vi "all filters coeffs.vi"(9 "taps diff":i32=17, 10 "sampling freq: fs":dbl=110250.0 min=-1e-308 max=1e+308 format="%0.2f", 11 "?":T2={"Amplitude"=1.0, "Lower Freq"=0.0, "Higher Freq"=25000.0, "Weighted\nRipple"=1e-06} {"Weighted\nRipple" min=-1e-308 max=1e+308 format="%0.2e"; "Higher Freq" min=-1e-308 max=1e+308 format="%0.2f"; "Lower Freq" min=-1e-308 max=1e+308 format="%0.2f"; "Amplitude" min=-1e-308 max=1e+308 format="%0.2f"}) -> (1 "ripple diff":dbl format="%0.2f", 2 "diff":dbl[](array[numeric])=[-1.090529051367417e-05, 0.00012379655057511986, -0.0007235759415153059, 0.0028997025258309344, -0.00899855784923205, 0.023414742171632856, -0.055622216670635403, 0.14563551285330884, 0.0, -0.14563551285330884, 0.055622216670635403, -0.023414742171632856, 0.00899855784923205, -0.0028997025258309344, 0.0007235759415153059, -0.00012379655057511986, 1.090529051367417e-05])   [LabVIEW 2017]
uses:
  <vilib>/Analysis/2dsp.llb/Real FFT.vi
  <vilib>/Analysis/3filter.llb/FIR Filter (DBL).vi
  <vilib>/Analysis/NI_AALBase.lvlib
  <vilib>/Analysis/NI_AALPro.lvlib
panel:
  in  "Tab Control":T1(tab)
  in  "?":T2={"Amplitude"=1.0, "Lower Freq"=1000.0, "Higher Freq"=49000.0, "Weighted\nRipple"=0.001} {"Weighted\nRipple" min=-1e-308 max=1e+308 format="%0.2e"; "Higher Freq" min=-1e-308 max=1e+308 format="%0.2f"; "Lower Freq" min=-1e-308 max=1e+308 format="%0.2f"; "Amplitude" min=-1e-308 max=1e+308 format="%0.2f"}
  in  "taps hilbert":i32=33
  in  "sampling freq: fs 2":dbl=110250.0 min=-1e-308 max=1e+308 format="%0.2f"
  out "hilbert":dbl[](graph)
  out "ripple hilbert":dbl format="%0.2f"
  out "hilbert":dbl[](array[numeric])
  out "K(omega) 2":dbl[](graph)
  out "diff":dbl[](graph)
  out "K(omega)":dbl[](graph)
  in  "demp":dbl=0.7
  in  "Fr":dbl=12000.0
  out "g1":dbl
  out "g2":dbl
  in  "discr freq":dbl=110250.0
  out "error":i32
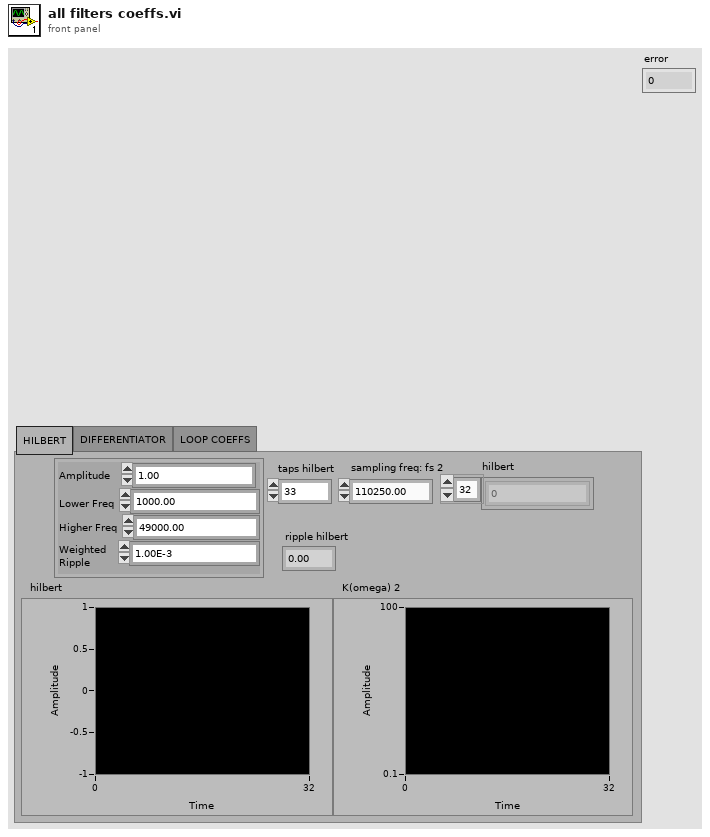
[diagram p1: front panel]
types:
  T1 = enum32{"HILBERT", "DIFFERENTIATOR", "LOOP COEFFS"}
  T2 = cluster{"Amplitude":dbl, "Lower Freq":dbl, "Higher Freq":dbl, "Weighted\nRipple":dbl}
  T3 = cluster{"Amplitude":dbl, "Lower Freq":dbl, "Higher Freq":dbl, "Weighted\nRipple":dbl}[]
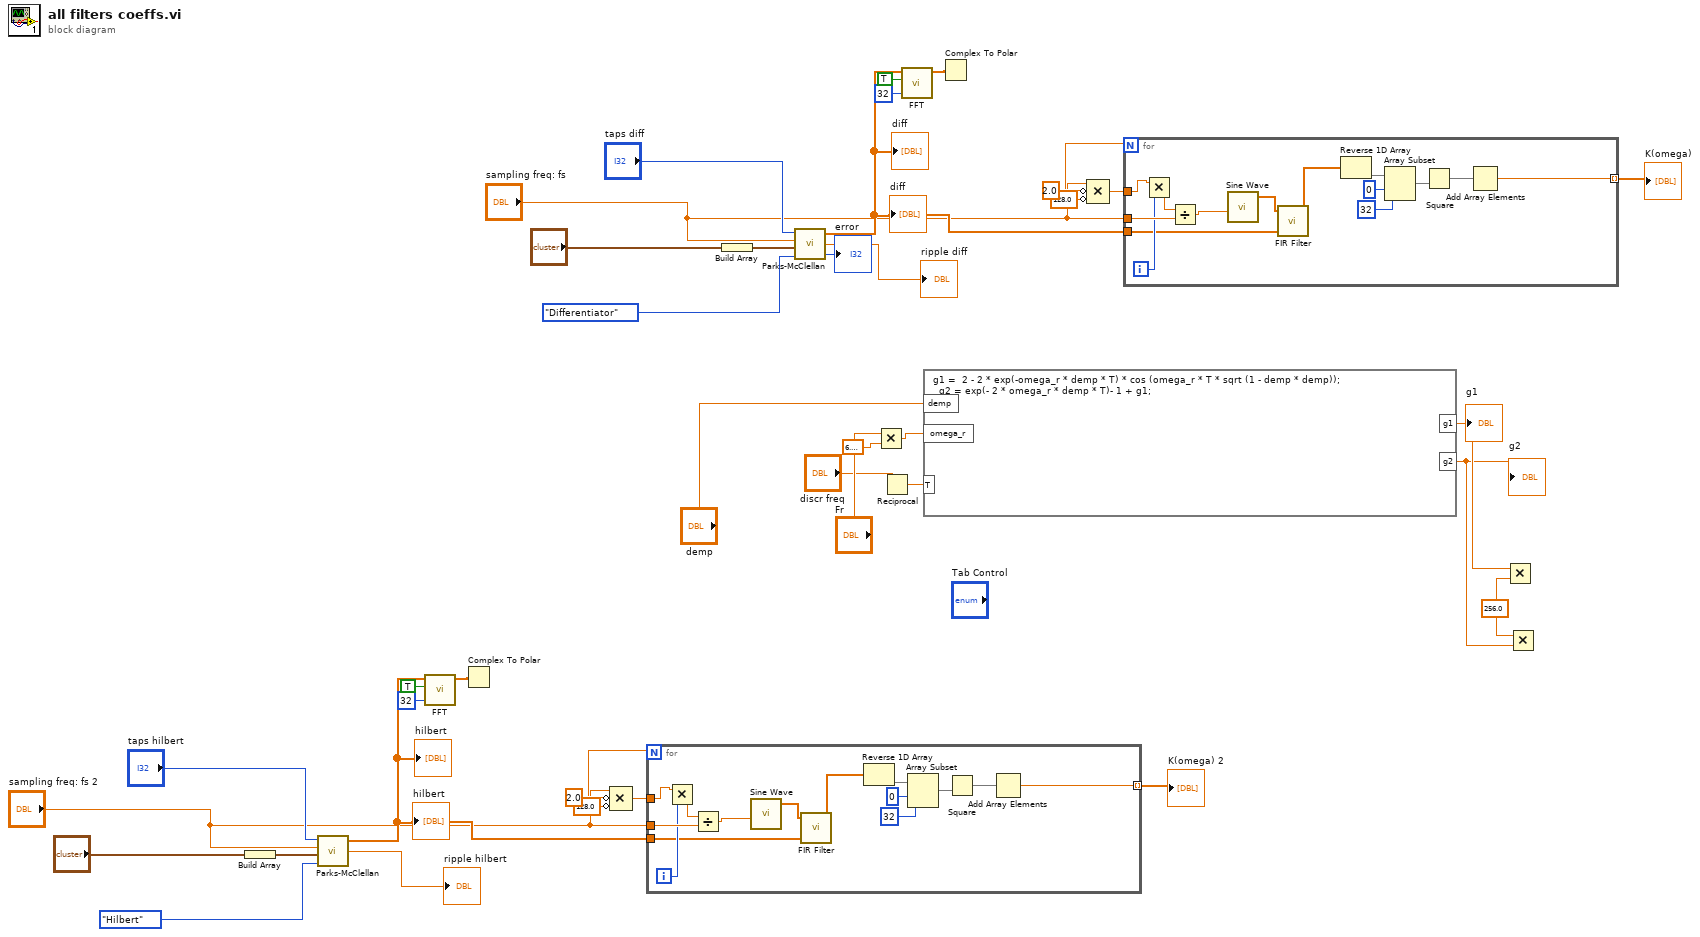
[diagram p0: block diagram]
diagram:
  w5 = 128.0 ("value")
  w17 = 256.0 ("y")
  w28 = 128.0 ("value")
  n1 = Build Array("?") -> (w13:T3)
  n2 = call <vilib>:"Parks-McClellan.vi"("filter type"=enum32{"Multiband", "Differentiator", "Hilbert"}."Hilbert", "Band Parameters"=w13, "sampling freq: fs"="sampling freq: fs 2", "# of taps"="taps hilbert") -> ("ripple"=→"ripple hilbert":dbl, "h"=w3:dbl[])  [unwired: 1 out]
  "hilbert" <- w3
  "hilbert" <- w3
  n3 = call-poly <vilib>:"FFT.vi"("FFT size"=32, "shift?"=TRUE, "X"=w3) -> ("FFT {X}"=w9:cdb[])  [unwired: 7 in, 1 out]
  n4 = Complex To Polar(r * e^(i*theta)=w9) -> ()  [unwired: 2 out]
  n5 = Compound Arithmetic op=MULTIPLY("sampling freq: fs 2", invert 2.0 ("y"), invert w5) -> (w4:dbl)
  n6 = for {
    N: w5 -> [_]
    tunnel: "sampling freq: fs 2" -> [w51]
    tunnel: w4 -> [w48]
    tunnel: w3 -> [w46]
    tunnel: [w39] -> w2 mode=indexing
    i -> [w49]
    n7 = Multiply(x=w48, y=w49) -> (x*y=w50:dbl)
    n8 = Divide(x=w50, y=w51) -> (x/y=w52:dbl)
    n9 = call <vilib>:"Sine Wave.vi"("frequency"=w52) -> ("sine wave"=w47:dbl[])  [unwired: 4 in, 2 out]
    n10 = call-poly <vilib>:"FIR Filter.vi"("FIR Coefficients"=w46, "X"=w47) -> ("Filtered X"=w44:dbl[])  [unwired: 2 in, 1 out]
    n11 = Reverse 1D Array(array=w44) -> (reversed array=w43:dbl[])
    n12 = Array Subset(array=w43, index=0, length=32) -> (w42:dbl[])
    n13 = Square(x=w42) -> (x^2=w45:dbl[])
    n14 = Add Array Elements(numeric array=w45) -> (sum=w39:dbl)
  }
  "K(omega) 2" <- w2
  n15 = Build Array("?") -> (w37:T3)
  n16 = call <vilib>:"Parks-McClellan.vi"("filter type"=enum32{"Multiband", "Differentiator", "Hilbert"}."Differentiator", "Band Parameters"=w37, "sampling freq: fs"="sampling freq: fs", "# of taps"="taps diff") -> ("error"=→"error":i32, "ripple"=→"ripple diff":dbl, "h"=w26:dbl[])
  "diff" <- w26
  "diff" <- w26
  n17 = Multiply(x="Fr", y=6.283185307179586) -> (x*y=w21:dbl)
  n18 = Reciprocal(x="discr freq") -> (1/x=w18:dbl)
  n19 = call-poly <vilib>:"FFT.vi"("FFT size"=32, "shift?"=TRUE, "X"=w26) -> ("FFT {X}"=w32:cdb[])  [unwired: 7 in, 1 out]
  n20 = formula code="g1 =  2 - 2 * exp(-omega_r * demp * T) * cos (omega_r * T * sqrt (1 - demp * demp));\n  g2 = exp(- 2 * omega_r * demp * T)- 1 + g1;"("demp"="demp", "omega_r"=w21, "T"=w18) -> ("g1"=w16:dbl, "g2"=w15:dbl)
  "g1" <- w16
  "g2" <- w15
  n21 = Complex To Polar(r * e^(i*theta)=w32) -> ()  [unwired: 2 out]
  n22 = Compound Arithmetic op=MULTIPLY("sampling freq: fs", invert 2.0 ("y"), invert w28) -> (w27:dbl)
  n23 = for {
    N: w28 -> [_]
    tunnel: "sampling freq: fs" -> [w65]
    tunnel: w27 -> [w62]
    tunnel: w26 -> [w60]
    tunnel: [w53] -> w25 mode=indexing
    i -> [w63]
    n24 = Multiply(x=w62, y=w63) -> (x*y=w64:dbl)
    n25 = Divide(x=w64, y=w65) -> (x/y=w66:dbl)
    n26 = call <vilib>:"Sine Wave.vi"("frequency"=w66) -> ("sine wave"=w61:dbl[])  [unwired: 4 in, 2 out]
    n27 = call-poly <vilib>:"FIR Filter.vi"("FIR Coefficients"=w60, "X"=w61) -> ("Filtered X"=w58:dbl[])  [unwired: 2 in, 1 out]
    n28 = Reverse 1D Array(array=w58) -> (reversed array=w57:dbl[])
    n29 = Array Subset(array=w57, index=0, length=32) -> (w56:dbl[])
    n30 = Square(x=w56) -> (x^2=w59:dbl[])
    n31 = Add Array Elements(numeric array=w59) -> (sum=w53:dbl)
  }
  "K(omega)" <- w25
  n32 = Multiply(x=w16, y=w17) -> ()  [unwired: 1 out]
  n33 = Multiply(x=w17, y=w15) -> ()  [unwired: 1 out]
